vi "XNET String To IO Name (LIN Schedule).vi"(3 "string":string) -> (0 "XNET LIN schedule":refnum<k21>)   [LabVIEW 2018]
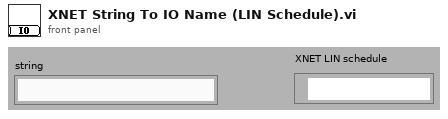
[diagram p1: front panel]
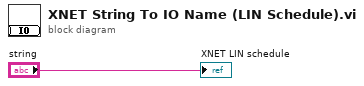
[diagram p0: block diagram]
diagram:
  "XNET LIN schedule" <- "string"
